vi "Build Self Test Switch String.vi"() -> ()   [LabVIEW 2010]
panel:
  out "String":string
  in  "Array":T1(array[cluster])
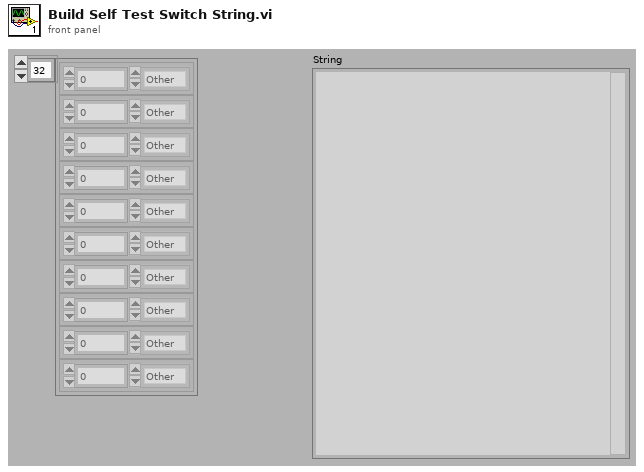
[diagram p1: front panel]
types:
  T1 = cluster{"Type":enum16{"Other", "Col27", "Col29", "Col31"}, "Channel":i32}[]
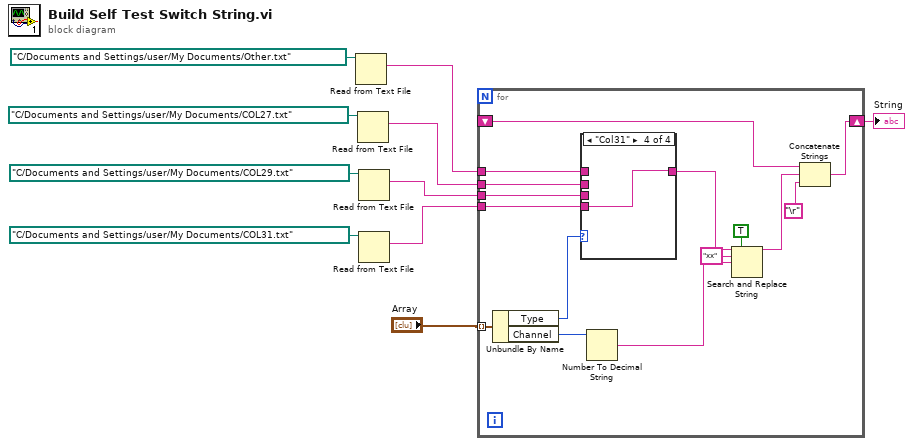
[diagram p0: block diagram]
diagram:
  n1 = Read from Text File(file (use dialog)=path "C:/Documents and Settings/user/My Documents/Other.txt") -> (text=w6:string)  [unwired: 3 in, 3 out]
  n2 = Read from Text File(file (use dialog)=path "C:/Documents and Settings/user/My Documents/COL27.txt") -> (text=w5:string)  [unwired: 3 in, 3 out]
  n3 = Read from Text File(file (use dialog)=path "C:/Documents and Settings/user/My Documents/COL29.txt") -> (text=w4:string)  [unwired: 3 in, 3 out]
  n4 = Read from Text File(file (use dialog)=path "C:/Documents and Settings/user/My Documents/COL31.txt") -> (text=w3:string)  [unwired: 3 in, 3 out]
  n5 = for {
    tunnel: w6 -> [w25]
    tunnel: w5 -> [w24]
    tunnel: w4 -> [w23]
    tunnel: w3 -> [w22]
    tunnel: "Array" -> [w21] mode=indexing
    shift-right: [w16] -> w1
    shift-left: _ -> [w17]
    n6 = Unbundle By Name(w21) -> ("Type"=w20:enum16{"Other", "Col27", "Col29", "Col31"}, "Channel"=w19:i32)
    n7 = case shown="\"Col31\"" w20 {
      tunnel: w25 -> [w26 _ _ _]
      tunnel: [w26 w27 w28 w29] -> w14
      tunnel: w24 -> [_ w27 _ _]
      tunnel: w23 -> [_ _ w28 _]
      tunnel: w22 -> [_ _ _ w29]
      frame "Other", Default {
      }
      frame "Col27" {
      }
      frame "Col29" {
      }
      frame "Col31" {
      }
    }
    n8 = Number To Decimal String(number=w19) -> (decimal integer string=w18:string)  [unwired: 1 in]
    n9 = Search and Replace String(replace all?=TRUE ("replace all? (F)"), input string=w14, search string="xx", replace string=w18) -> (result string=w15:string)  [unwired: 4 in, 3 out]
    n10 = Concatenate Strings(w17, w15, "\r") -> (w16:string)
  }
  "String" <- w1
